vi "rsscope_core_global.vi"() -> ()   [LabVIEW 2018] (continued)
the firmware version that is currently installed on the instrument.\n\nAvailable Repeated Capabilities:\nNone\n\nRemote-control command(s):\nDIAGnostic:SERVice:FWVersion?"}, {"Level"=2, "Class Only"=FALSE, "Identifier"="RSSCOPE_ATTR_COMPUTER_NAME", "Descriptive Name"="Computer Name", "Data Type"=2, "Command"="DIAG:SERV:COMP", "Access"=2, "Range Table"="", "Read Callback"="", "Write Callback"="", "Supported Models"="", "Instrument Options"="", "Flags"=0, "Help"="Configures the computer name that is currently defined. The computer name is required when configuring a network.\n\nAvailable Repeated Capabilities:\nNone\n\nRemote-control command(s):\nDIAGnostic:SERVice:COMPutername"}, {"Level"=2, "Class Only"=FALSE, "Identifier"="RSSCOPE_ATTR_MATERIAL_NUMBER", "Descriptive Name"="Material Number", "Data Type"=2, "Command"="DIAG:SERV:PART?", "Access"=0, "Range Table"="", "Read Callback"="", "Write Callback"="", "Supported Models"="", "Instrument Options"="", "Flags"=0, "Help"="Configures the material number of your instrument. This number is required to order a new option, and in case of service.\n\nAvailable Repeated Capabilities:\nNone\n\nRemote-control command(s):\nDIAGnostic:SERVice:PARTnumber?"}, {"Level"=2, "Class Only"=FALSE, "Identifier"="RSSCOPE_ATTR_SERIAL_NUMBER", "Descriptive Name"="Serial Number", "Data Type"=2, "Command"="DIAG:SERV:SER?", "Access"=0, "Range Table"="", "Read Callback"="", "Write Callback"="", "Supported Models"="", "Instrument Options"="", "Flags"=0, "Help"="Returns the serial number of your instrument. This number is required to order a new option, and in case of service.\n\nAvailable Repeated Capabilities:\nNone\n\nRemote-control command(s):\nDIAGnostic:SERVice:SERialnumber?"}, {"Level"=2, "Class Only"=FALSE, "Identifier"="RSSCOPE_ATTR_START_SELFTEST", "Descriptive Name"="Start Selftest", "Data Type"=4, "Command"="DIAG:SERV:STST:EXEC", "Access"=1, "Range Table"="", "Read Callback"="", "Write Callback"="", "Supported Models"="", "Instrument Options"="", "Flags"=0, "Help"="Starts the selftest.\n\nAvailable Repeated Capabilities:\nNone\n\nRemote-control command(s):\nDIAGnostic:SERVice:STST:EXECute"}, {"Level"=2, "Class Only"=FALSE, "Identifier"="RSSCOPE_ATTR_SELFTEST_STATUS", "Descriptive Name"="Selftest Status", "Data Type"=0, "Command"="DIAG:SERV:STST:STAT?", "Access"=0, "Range Table"="rsscope_rngSelftestStatus", "Read Callback"="", "Write Callback"="", "Supported Models"="", "Instrument Options"="", "Flags"=0, "Help"="Returns the summary result of the selftest.\n\nAvailable Repeated Capabilities:\nNone\n\nRemote-control command(s):\nDIAGnostic:SERVice:STST:STATe?"}, {"Level"=2, "Class Only"=FALSE, "Identifier"="RSSCOPE_ATTR_SET_QUERY_PATTERN_FORMAT", "Descriptive Name"="Set Query Pattern Format", "Data Type"=0, "Command"="FORM:BPAT", "Access"=2, "Range Table"="rsscope_rngPatternFormat", "Read Callback"="", "Write Callback"="", "Supported Models"="", "Instrument Options"="", "Flags"=0, "Help"="Configures the format for all bit pattern queries.\n\nAvailable Repeated Capabilities:\nNone\n\nRemote-control command(s):\nFORMat:BPATtern"}, {"Level"=2, "Class Only"=FALSE, "Identifier"="RSSCOPE_ATTR_SERVICE_MODE_PASSWORD", "Descriptive Name"="Service Mode Password", "Data Type"=2, "Command"="DIAG:SERV:PWD", "Access"=1, "Range Table"="", "Read Callback"="", "Write Callback"="", "Supported Models"="", "Instrument Options"="", "Flags"=0, "Help"="Sets the password to enter the service mode.\n\nAvailable Repeated Capabilities:\nNone\n\nRemote-control command(s):\nDIAGnostic:SERVice:PWD"}, {"Level"=2, "Class Only"=FALSE, "Identifier"="RSSCOPE_ATTR_SCOPE_MODEL", "Descriptive Name"="Scope Model", "Data Type"=0, "Command"="DIAG:SERV:WFAM?", "Access"=0, "Range Table"="RsScope_rngScopeModel", "Read Callback"="", "Write Callback"="", "Supported Models"="", "Instrument Options"="", "Flags"=0, "Help"="Returns the model name of the oscilloscope.\n\nAvailable Repeated Capabilities:\nNone\n\nRemote-control command(s):\nDIAGnostic:SERVice:WFAModel?"}, {"Level"=2, "Class Only"=FALSE, "Identifier"="RSSCOPE_ATTR_SCOPE_SERIES", "Descriptive Name"="Scope Series", "Data Type"=0, "Command"="DIAG:SERV:WFAS?", "Access"=0, "Range Table"="RsScope_rngScopeSeries", "Read Callback"="", "Write Callback"="", "Supported Models"="", "Instrument Options"="", "Flags"=0, "Help"="Returns the model series of the oscilloscope.\n\nAvailable Repeated Capabilities:\nNone\n\nRemote-control command(s):\nDIAGnostic:SERVice:WFASeries?"}, {"Level"=2, "Class Only"=FALSE, "Identifier"="RSSCOPE_ATTR_SCOPE_FAMILY", "Descriptive Name"="Scope Family", "Data Type"=0, "Command"="DIAG:SERV:WFAT?", "Access"=0, "Range Table"="RsScope_rngScopeFamily", "Read Callback"="", "Write Callback"="", "Supported Models"="", "Instrument Options"="", "Flags"=0, "Help"="Returns the instrument family of the oscilloscope.\n\nAvailable Repeated Capabilities:\nNone\n\nRemote-control command(s):\nDIAGnostic:SERVice:WFAType?"}, {"Level"=1, "Class Only"=TRUE, "Identifier"="", "Descriptive Name"="Utility Functions", "Data Type"=0, "Command"="", "Access"=0, "Range Table"="", "Read Callback"="", "Write Callback"="", "Supported Models"="", "Instrument Options"="", "Flags"=0, "Help"="Utility attributes and functions."}, {"Level"=2, "Class Only"=FALSE, "Identifier"="RSSCOPE_ATTR_CALIBRATION", "Descriptive Name"="Calibration", "Data Type"=0, "Command"="*CAL?", "Access"=0, "Range Table"="", "Read Callback"="", "Write Callback"="", "Supported Models"="", "Instrument Options"="", "Flags"=0, "Help"="Initiates a calibration of the instrument and subsequently queries the calibration status. Responses > 0 indicate errors.\n\nAvailable Repeated Capabilities:\nNone\n\nRemote-control command(s):\n*CAL?"}, {"Level"=2, "Class Only"=FALSE, "Identifier"="RSSCOPE_ATTR_SELF_TEST_QUERY", "Descriptive Name"="Self-Test Query", "Data Type"=0, "Command"="*TST?", "Access"=0, "Range Table"="", "Read Callback"="", "Write Callback"="", "Supported Models"="", "Instrument Options"="", "Flags"=1, "Help"="Triggers selftests of the instrument and returns an error code in decimal form (see Service Manual supplied with the instrument). &apos;0&apos; indicates no errors occured.\n\nAvailable Repeated Capabilities:\nNone\n\nRemote-control command(s):\n*TST?"}, {"Level"=2, "Class Only"=FALSE, "Identifier"="RSSCOPE_ATTR_BYTE_ORDER", "Descriptive Name"="Byte Order", "Data Type"=0, "Command"="FORM:BORD", "Access"=2, "Range Table"="rsscope_rngByteOrder", "Read Callback"="", "Write Callback"="", "Supported Models"="", "Instrument Options"="", "Flags"=0, "Help"="Sets the endianess.\n\nAvailable Repeated Capabilities:\nNone\n\nRemote-control command(s):\nFORMat:BORDer"}, {"Level"=2, "Class Only"=FALSE, "Identifier"="RSSCOPE_ATTR_SYSTEM_ERROR_ALL", "Descriptive Name"="System Error All", "Data Type"=2, "Command"="SYST:ERR:ALL?", "Access"=0, "Range Table"="", "Read Callback"="", "Write Callback"="", "Supported Models"="", "Instrument Options"="", "Flags"=0, "Help"="Queries the error/event queue for all unread items and removes them from the queue. The response is a comma-separated list of error number and a short description of the error in FIFO order.\nPositive error numbers are instrument-dependent. Negative error numbers are reserved by the SCPI standard.\n\nAvailable Repeated Capabilities:\nNone\n\nRemote-control command(s):\nSYSTem:ERRor:ALL?"}, {"Level"=2, "Class Only"=FALSE, "Identifier"="RSSCOPE_ATTR_SYSTEM_ERROR", "Descriptive Name"="System Error", "Data Type"=2, "Command"="SYST:ERR?", "Access"=0, "Range Table"="", "Read Callback"="", "Write Callback"="", "Supported Models"="", "Instrument Options"="", "Flags"=0, "Help"="Queries error from error queue.\n\nAvailable Repeated Capabilities:\nNone\n\nRemote-control command(s):\nSYSTem:ERRor?"}, {"Level"=2, "Class Only"=FALSE, "Identifier"="RSSCOPE_ATTR_SYSTEM_ERROR_CODE_ALL", "Descriptive Name"="System Error Code All", "Data Type"=2, "Command"="SYST:ERR:CODE:ALL?", "Access"=0, "Range Table"="", "Read Callback"="", "Write Callback"="", "Supported Models"="", "Instrument Options"="", "Flags"=0, "Help"="Queries the error/event queue for all unread items and removes them from the queue. The response is a comma separated list of error numbers in FIFO order. Positive error numbers are instrument-dependent. Negative error numbers are reserved by the SCPI standard.\n\nAvailable Repeated Capabilities:\nNone\n\nRemote-control command(s):\nSYSTem:ERRor:CODE:ALL?"}, {"Level"=2, "Class Only"=FALSE, "Identifier"="RSSCOPE_ATTR_SYSTEM_ERROR_CODE", "Descriptive Name"="System Error Code", "Data Type"=0, "Command"="SYST:ERR:CODE?", "Access"=0, "Range Table"="", "Read Callback"="", "Write Callback"="", "Supported Models"="", "Instrument Options"="", "Flags"=0, "Help"="Queries the error/event queue for the oldest item and removes it from the queue. The response is the error number. Positive error numbers are instrument-dependent. Negative error numbers are reserved by the SCPI standard.\n\nAvailable Repeated Capabilities:\nNone\n\nRemote-control command(s):\nSYSTem:ERRor:CODE[:NEXT]?"}, {"Level"=2, "Class Only"=FALSE, "Identifier"="RSSCOPE_ATTR_SYSTEM_ERROR_COUNT", "Descriptive Name"="System Error Count", "Data Type"=0, "Command"="SYST:ERR:COUN?", "Access"=0, "Range Table"="", "Read Callback"="", "Write Callback"="", "Supported Models"="", "Instrument Options"="", "Flags"=0, "Help"="Queries the number of entries in the error queue.\n\nAvailable Repeated Capabilities:\nNone\n\nRemote-control command(s):\nSYSTem:ERRor:COUNt?"}, {"Level"=2, "Class Only"=FALSE, "Identifier"="RSSCOPE_ATTR_OPERATION_REGISTER_ENABLED", "Descriptive Name"="Operation Register Enabled", "Data Type"=0, "Command"="STAT:OPER:ENAB", "Access"=2, "Range Table"="RsScope_rngRegister", "Read Callback"="", "Write Callback"="", "Supported Models"="", "Instrument Options"="", "Flags"=0, "Help"="Controls the ENABle part of the STATus:OPERation register. The ENABle defines which events in the EVENt part of the status register are forwarded to the OPERation summary bit (bit 7) of the status byte. The status byte can be used to create a service request.\n\nAvailable Repeated Capabilities:\nNone\n\nRemote-control command(s):\nSTATus:OPERation:ENABle"}, {"Level"=2, "Class Only"=FALSE, "Identifier"="RSSCOPE_ATTR_OPERATION_REGISTER_EVENT", "Descriptive Name"="Operation Register Event", "Data Type"=0, "Command"="STAT:OPER?", "Access"=0, "Range Table"="", "Read Callback"="", "Write Callback"="", "Supported Models"="", "Instrument Options"="", "Flags"=0, "Help"="Attribute returns information on actions the instrument has executed since the last reading. Reading the EVENt register deletes its contents.\nBits:\n0 = ALIGnment\n2 = AUToset\n3= WTRIgger (wait for trigger)\n4= MEASuring\n\nAvailable Repeated Capabilities:\nNone\n\nRemote-control command(s):\nSTATus:OPERation[:EVENt]?"}, {"Level"=2, "Class Only"=FALSE, "Identifier"="RSSCOPE_ATTR_PROCESS_ALL_PREVIOUS_COMMANDS", "Descriptive Name"="Process All Previous Commands", "Data Type"=4, "Command"="*WAI", "Access"=1, "Range Table"="", "Read Callback"="", "Write Callback"="", "Supported Models"="", "Instrument Options"="", "Flags"=2, "Help"="Stops further command processing until all commands sent before *WAI have been executed.\n\nAvailable Repeated Capabilities:\nNone\n\nRemote-control command(s):\n*WAI"}, {"Level"=2, "Class Only"=FALSE, "Identifier"="RSSCOPE_ATTR_GPIB_ADDRESS", "Descriptive Name"="GPIB Address", "Data Type"=0, "Command"="GPIB:ADDR", "Access"=2, "Range Table"="RsScope_rngGPIBAddress", "Read Callback"="", "Write Callback"="", "Supported Models"="", "Instrument Options"="", "Flags"=0, "Help"="Sets the GPIB address of the instrument. Changing the address has major effects on the communication to the remote computer.\n\nAvailable Repeated Capabilities:\nNone\n\nRemote-control command(s):\nGPIB:ADDRess"}, {"Level"=2, "Class Only"=FALSE, "Identifier"="RSSCOPE_ATTR_GPIB_TERMINATOR", "Descriptive Name"="GPIB Terminator", "Data Type"=0, "Command"="GPIB:TERM", "Access"=2, "Range Table"="RsScope_rngGPIBTerminator", "Read Callback"="", "Write Callback"="", "Supported Models"="", "Instrument Options"="", "Flags"=0, "Help"="Specifies the symbol that is used as a terminator in GPIB communication.\n\nAvailable Repeated Capabilities:\nNone\n\nRemote-control command(s):\nGPIB:TERMinator"}, {"Level"=2, "Class Only"=FALSE, "Identifier"="RSSCOPE_ATTR_SYSTEM_SHUTDOWN", "Descriptive Name"="System Shutdown", "Data Type"=4, "Command"="SYST:SHUT", "Access"=1, "Range Table"="", "Read Callback"="", "Write Callback"="", "Supported Models"="", "Instrument Options"="", "Flags"=0, "Help"="Starts the shutdown of the instrument (firmware and operating system).\n\nAvailable Repeated Capabilities:\nNone\n\nRemote-control command(s):\nSYSTem:SHUTdown"}, {"Level"=2, "Class Only"=FALSE, "Identifier"="RSSCOPE_ATTR_SYSTEM_VERSION", "Descriptive Name"="System Version", "Data Type"=2, "Command"="SYST:VERS?", "Access"=0, "Range Table"="", "Read Callback"="", "Write Callback"="", "Supported Models"="", "Instrument Options"="", "Flags"=0, "Help"="Queries the SCPI version number to which the instrument complies. The instrument complies to the final SCPI version 1999.0.\n\nAvailable Repeated Capabilities:\nNone\n\nRemote-control command(s):\nSYSTem:VERSion?"}, {"Level"=2, "Class Only"=FALSE, "Identifier"="RSSCOPE_ATTR_SYSTEM_PRESET", "Descriptive Name"="System Preset", "Data Type"=4, "Command"="SYST:PRES", "Access"=1, "Range Table"="", "Read Callback"="", "Write Callback"="", "Supported Models"="", "Instrument Options"="", "Flags"=0, "Help"="Resets the instrument to the factory default settings, to the initial state. Factory settings comprise all instrument settings, including display, intensity and transparency settings. After loading factory defaults, perform a self-aligment to synchronize the signal data.\n\nAvailable Repeated Capabilities:\nNone\n\nRemote-control command(s):\nSYSTem:PRESet"}, {"Level"=2, "Class Only"=FALSE, "Identifier"="RSSCOPE_ATTR_SYSTEM_DEVICE_ID", "Descriptive Name"="System Device ID", "Data Type"=2, "Command"="SYST:DEV:ID?", "Access"=0, "Range Table"="", "Read Callback"="", "Write Callback"="", "Supported Models"="", "Instrument Options"="", "Flags"=0, "Help"="Returns the instrument ID - that is the material number and the serial number.\n\nAvailable Repeated Capabilities:\nNone\n\nRemote-control command(s):\nSYSTem:DEVice:ID?"}, {"Level"=2, "Class Only"=FALSE, "Identifier"="RSSCOPE_ATTR_LOCK_LOCAL_KEYS", "Descriptive Name"="Lock Local Keys", "Data Type"=3, "Command"="SYST:KLOC", "Access"=2, "Range Table"="", "Read Callback"="", "Write Callback"="", "Supported Models"="", "Instrument Options"="", "Flags"=0, "Help"="Locks or unlocks the local controls of the instrument. This includes the front panel keys, the keyboard, or other local interfaces. except for the &apos;View&apos; button on the display.\n\nAvailable Repeated Capabilities:\nNone\n\nRemote-control command(s):\nSYSTem:KLOCk"}, {"Level"=2, "Class Only"=FALSE, "Identifier"="RSSCOPE_ATTR_SYSTEM_INFO_DEVICE_FOOTPRINT", "Descriptive Name"="System Info Device Footprint", "Data Type"=2, "Command"="SYST:DFPR", "Access"=2, "Range Table"="", "Read Callback"="", "Write Callback"="", "Supported Models"="", "Instrument Options"="", "Flags"=0, "Help"="The device footprint contains the configuration of the instrument, installed modules, installed software and software licenses. This information is written in the device footprint xml file might be useful in case of maintenance or support request.\nThe query returns the information as block data. The setting command saves the device footprint xml file in the specified path.\nIt is also possible to access the device footprint xml file via the instrument&apos;s web browser. Therefore, the directory containing the xml file must be enabled for sharing.\n\nAvailable Repeated Capabilities:\nNone\n\nRemote-control command(s):\nSYSTem:DFPRint"}, {"Level"=2, "Class Only"=FALSE, "Identifier"="RSSCOPE_ATTR_SYSTEM_REMOTE_CONTROL_COMMAND_SET", "Descriptive Name"="System Remote Control Command Set", "Data Type"=2, "Command"="SYST:LANG", "Access"=2, "Range Table"="", "Read Callback"="", "Write Callback"="", "Supported Models"="", "Instrument Options"="", "Flags"=0, "Help"="Defines the remote control behavior of the instrument and sets the remote control command set.\n\nAvailable Repeated Capabilities:\nNone\n\nRemote-control command(s):\nSYSTem:LANGuage"}, {"Level"=2, "Class Only"=FALSE, "Identifier"="RSSCOPE_ATTR_QUERY_SYSTEM_DATE", "Descriptive Name"="Query System Date", "Data Type"=2, "Command"="SYST:DATE?", "Access"=0, "Range Table"="", "Read Callback"="", "Write Callback"="", "Supported Models"="", "Instrument Options"="", "Flags"=0, "Help"="Returns the date of the internal calendar. String is in the format &apos;<Year>,<Month>,<Day>&apos;.\n\nAvailable Repeated Capabilities:\nNone\n\nRemote-control command(s):\nSYSTem:DATE?"}, {"Level"=2, "Class Only"=FALSE, "Identifier"="RSSCOPE_ATTR_QUERY_SYSTEM_TIME", "Descriptive Name"="Query System Time", "Data Type"=2, "Command"="SYST:TIME?", "Access"=0, "Range Table"="", "Read Callback"="", "Write Callback"="", "Supported Models"="", "Instrument Options"="", "Flags"=0, "Help"="Returns the UTC (Universal Time Coordinated) of the internal clock. To define the current local time, use the time zone setting of the operating system (Setup > Time, date). Return string is of the format &apos;<Hour>,<Minute>,<Second>&apos;.\n\nAvailable Repeated Capabilities:\nNone\n\nRemote-control command(s):\nSYSTem:TIME?"}, {"Level"=2, "Class Only"=TRUE, "Identifier"="", "Descriptive Name"="Remote Trace", "Data Type"=0, "Command"="", "Access"=0, "Range Table"="", "Read Callback"="", "Write Callback"="", "Supported Models"="", "Instrument Options"="", "Flags"=0, "Help"="The attributes and functions in this section configure tracing of the remote control interface and of events. They also configure the display of the SCPI remote trace."}, {"Level"=3, "Class Only"=FALSE, "Identifier"="RSSCOPE_ATTR_REMOTE_TRACE_FILE_NAME", "Descriptive Name"="Remote Trace File Name", "Data Type"=2, "Command"="TRAC:REM:MODE:FILE:NAME", "Access"=2, "Range Table"="", "Read Callback"="", "Write Callback"="", "Supported Models"="", "Instrument Options"="", "Flags"=0, "Help"="Sets the directory and file name where the remote trace file is stored.\n\nAvailable Repeated Capabilities:\nNone\n\nRemote-control command(s):\nTRACe:REMote:MODE:FILE:NAME"}, {"Level"=3, "Class Only"=FALSE, "Identifier"="RSSCOPE_ATTR_REMOTE_TRACE_FILE_FORMAT", "Descriptive Name"="Remote Trace File Format", "Data Type"=0, "Command"="TRAC:REM:MODE:FILE:FORM", "Access"=2, "Range Table"="RsScope_rngRemoteTraceFileFormat", "Read Callback"="", "Write Callback"="", "Supported Models"="", "Instrument Options"="", "Flags"=0, "Help"="Sets the file format of the remote trace file.\n\nAvailable Repeated Capabilities:\nNone\n\nRemote-control command(s):\nTRACe:REMote:MODE:FILE:FORMat"}, {"Level"=3, "Class Only"=FALSE, "Identifier"="RSSCOPE_ATTR_REMOTE_TRACE_FILE_SIZE", "Descriptive Name"="Remote Trace File Size", "Data Type"=0, "Command"="TRAC:REM:MODE:FILE:SIZE", "Access"=2, "Range Table"="", "Read Callback"="", "Write Callback"="", "Supported Models"="", "Instrument Options"="", "Flags"=0, "Help"="Sets the maximum size of the remote trace file.\n\nAvailable Repeated Capabilities:\nNone\n\nRemote-control command(s):\nTRACe:REMote:MODE:FILE:SIZE"}, {"Level"=3, "Class Only"=FALSE, "Identifier"="RSSCOPE_ATTR_REMOTE_TRACE_START_MODE", "Descriptive Name"="Remote Trace Start Mode", "Data Type"=0, "Command"="TRAC:REM:MODE:FILE:STAR", "Access"=2, "Range Table"="RsScope_rngStartMode", "Read Callback"="", "Write Callback"="", "Supported Models"="", "Instrument Options"="", "Flags"=0, "Help"="Defines how the remote trace is started.\n\nAvailable Repeated Capabilities:\nNone\n\nRemote-control command(s):\nTRACe:REMote:MODE:FILE:STARtmode"}, {"Level"=3, "Class Only"=FALSE, "Identifier"="RSSCOPE_ATTR_REMOTE_TRACE_STOP_MODE", "Descriptive Name"="Remote Trace Stop Mode", "Data Type"=0, "Command"="TRAC:REM:MODE:FILE:STOP", "Access"=2, "Range Table"="RsScope_rngStopMode", "Read Callback"="", "Write Callback"="", "Supported Models"="", "Instrument Options"="", "Flags"=0, "Help"="Defines when the remote trace is stopped.\n\nAvailable Repeated Capabilities:\nNone\n\nRemote-control command(s):\nTRACe:REMote:MODE:FILE:STOPmode"}, {"Level"=3, "Class Only"=FALSE, "Identifier"="RSSCOPE_ATTR_REMOTE_TRACE_ENABLED", "Descriptive Name"="Remote Trace Enabled", "Data Type"=3, "Command"="TRAC:REM:MODE:FILE:ENAB", "Access"=2, "Range Table"="", "Read Callback"="", "Write Callback"="", "Supported Models"="", "Instrument Options"="", "Flags"=0, "Help"="Enables and disables the remote trace to file.\n\nAvailable Repeated Capabilities:\nNone\n\nRemote-control command(s):\nTRACe:REMote:MODE:FILE:ENABle"}, {"Level"=3, "Class Only"=FALSE, "Identifier"="RSSCOPE_ATTR_REMOTE_TRACE_COMMAND_EXECUTION_DURATION_ENABLED", "Descriptive Name"="Remote Trace Command Execution Duration Enabled", "Data Type"=3, "Command"="TRAC:REM:MODE:FILE:DEX:DUR", "Access"=2, "Range Table"="", "Read Callback"="", "Write Callback"="", "Supported Models"="", "Instrument Options"="", "Flags"=0, "Help"="Traces the device execution time of a command.\n\nAvailable Repeated Capabilities:\nNone\n\nRemote-control command(s):\nTRACe:REMote:MODE:FILE:DEXecution:DURation"}, {"Level"=3, "Class Only"=FALSE, "Identifier"="RSSCOPE_ATTR_REMOTE_TRACE_RPC_OUTPUT_ENABLED", "Descriptive Name"="Remote Trace RPC Output Enabled", "Data Type"=3, "Command"="TRAC:REM:MODE:FILE:RPC", "Access"=2, "Range Table"="", "Read Callback"="", "Write Callback"="", "Supported Models"="", "Instrument Options"="", "Flags"=0, "Help"="Enables and disables output of rpc calls to remote trace.\n\nAvailable Repeated Capabilities:\nNone\n\nRemote-control command(s):\nTRACe:REMote:MODE:FILE:RPC"}, {"Level"=3, "Class Only"=FALSE, "Identifier"="RSSCOPE_ATTR_REMOTE_TRACE_PARSER_TRANSITIONS_OUTPUT_ENABLED", "Descriptive Name"="Remote Trace Parser Transitions Output Enabled", "Data Type"=3, "Command"="TRAC:REM:MODE:FILE:PARS", "Access"=2, "Range Table"="", "Read Callback"="", "Write Callback"="", "Supported Models"="", "Instrument Options"="", "Flags"=0, "Help"="Enables and disables output of parser transitions to remote trace.\n\nAvailable Repeated Capabilities:\nNone\n\nRemote-control command(s):\nTRACe:REMote:MODE:FILE:PARSer"}, {"Level"=3, "Class Only"=FALSE, "Identifier"="RSSCOPE_ATTR_REMOTE_TRACE_FUNCTION_NAMES_OUTPUT_ENABLED", "Descriptive Name"="Remote Trace Function Names Output Enabled", "Data Type"=3, "Command"="TRAC:REM:MODE:FILE:FUNC", "Access"=2, "Range Table"="", "Read Callback"="", "Write Callback"="", "Supported Models"="", "Instrument Options"="", "Flags"=0, "Help"="Enables and disables output of function names to remote trace.\n\nAvailable Repeated Capabilities:\nNone\n\nRemote-control command(s):\nTRACe:REMote:MODE:FILE:FUNCtions"}] {"Flags" format="%08b"; "Access" items=["Read Only", "Write Only", "Read/Write"]; "Data Type" items=["Integer 32", "Double", "String", "Boolean", "None", "Integer 64", "RawString"]}
  in  "Supported Models":string[](array[string])=["RTO", "RTE", "RTP"]
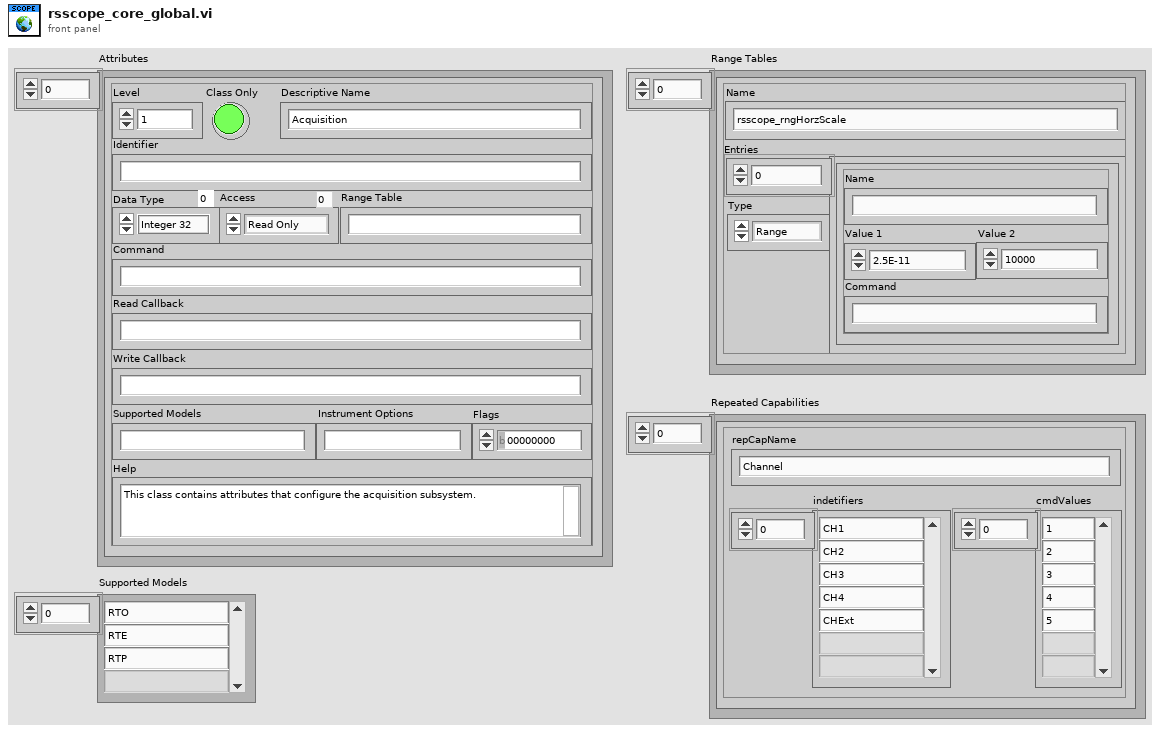
[diagram p1: front panel]
types:
  T1 = typedef "rsscope_rsidr_core.lvlib/type_Input_Format_RepCap.ctl" = cluster{"repCapName":string, "indetifiers":string[], "cmdValues":string[]}
  T2 = typedef "rsscope_rsidr_core.lvlib/type_Input_Format_RangeTable.ctl" = cluster{"Type":u16, "Name":string, "Entries":cluster{"Name":string, "Value 1":dbl, "Value 2":dbl, "Command":string}[]}
  T3 = typedef "rsscope_rsidr_core.lvlib/type_Input_Format_Attribute.ctl" = cluster{"Level":i32, "Class Only":bool, "Identifier":string, "Descriptive Name":string, "Data Type":u16, "Command":string, "Access":u16, "Range Table":string, "Read Callback":string, "Write Callback":string, "Supported Models":string, "Instrument Options":string, "Flags":i32, "Help":string}
diagram:
